vi "Actor Core.vi"(8 "error in":errorcluster, 11 "ViewableChart In":refnum<class "ViewableStatusBar.lvclass">) -> (0 "error out":errorcluster, 3 "Actor out":refnum<class "Actor.lvclass">)   [LabVIEW 2017, in "ViewableStatusBar.lvclass"]
doc: "(<B>Filename</B>: Actor Framework.lvlib:Actor.lvclass:Actor Core.vi)\n\nReceives messages to the actor, reacts to them, and initiates any error handling that may shut the actor down.\n\nDescendant classes may override this VI to append parallel tasks for the actor to complete while it handles messages. Overrides use the Call Parent Method node.\n\n<License>\nCopyright © 2017 Composed Systems, LLC | All rights reserved\nwww.composed.io\n\nAuthor: Ethan Stern <ethan.stern@composed.io>\n\nThis software is provided \"AS IS\" WITHOUT WARRANTIES, either express or implied, AND IS FOR EDUCATIONAL PURPOSES ONLY.\n</License>MVA Framework 1.7.0.33\nEthan Stern - Composed Systems\nCopyright (c) 2018, Composed Systems"
uses:
  ViewableStatusBar.lvclass
  C:/Program Files/National Instruments/LabVIEW 2017/vi.lib/Composed/GPM Packages/mva-framework/Source/Framework/IViewable/IViewable/IViewable.lvclass
  <vilib>/ActorFramework/Actor/Actor.lvclass
  mva-viewable/Source/IViewable/IViewable/IViewable.lvclass
panel:
  out "Status":string
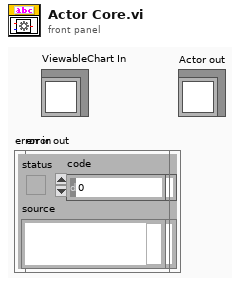
[diagram p1: front panel]
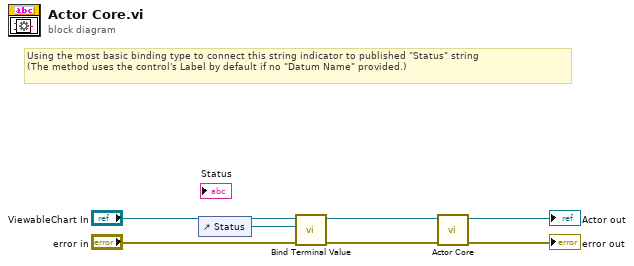
[diagram p0: block diagram]
diagram:
  # "Using the most basic binding type to connect this string indicator to published \"Status\" string\n(The method uses the control's Label by default if no \"Datum Name\" provided.)"
  n1 = control-ref of="Status"() -> (w1:refnum<vi>)
  n2 = call "Bind Terminal Value.vi"("error in (no error)"="error in", "Ctl Refnum"=w1, "IViewable in"="ViewableChart In") -> ("error out"=w2:errorcluster, "IViewable out"=w4:refnum<class "ViewableStatusBar.lvclass">)  [unwired: 7 in]
  n3 = call-parent "Actor Core.vi"("error in"=w2, "IViewable In"=w4) -> ("error out"=→"error out":errorcluster, "Actor out"=→"Actor out":refnum<class "Actor.lvclass">)  [unwired: 8 in]
